vi "Window-Error message.vi"(8 "error in (no error)":errorcluster, 11 "Message":string) -> (0 "Error Out (no error)":errorcluster)   [LabVIEW 2020]
doc: "Use this template to create a dialog box with event handling."
uses:
  <vilib>/Utility/error.llb/DialogType.ctl
  miscelaneous/Error window positioning/Error window pos FGV states.ctl
  Global Variables/General Globals.vi
panel:
  out "Message":string
  in  "Close":bool
  in  "Vertical Stop Button":bool
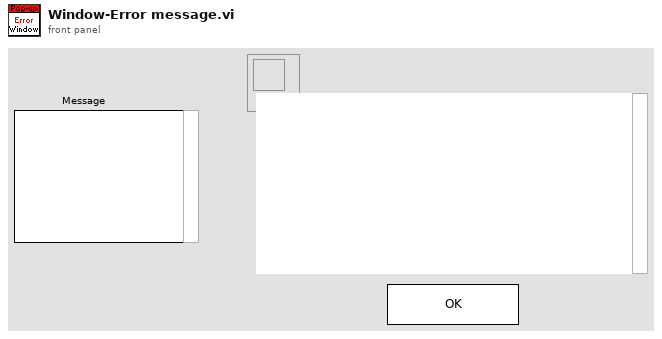
[diagram p1: front panel]
types:
  T1 = typedef "Error window pos FGV states.ctl" = enum16{"Read", "Window closed", "Window opened", "Reset"}
  T2 = typedef "DialogType.ctl" = u16
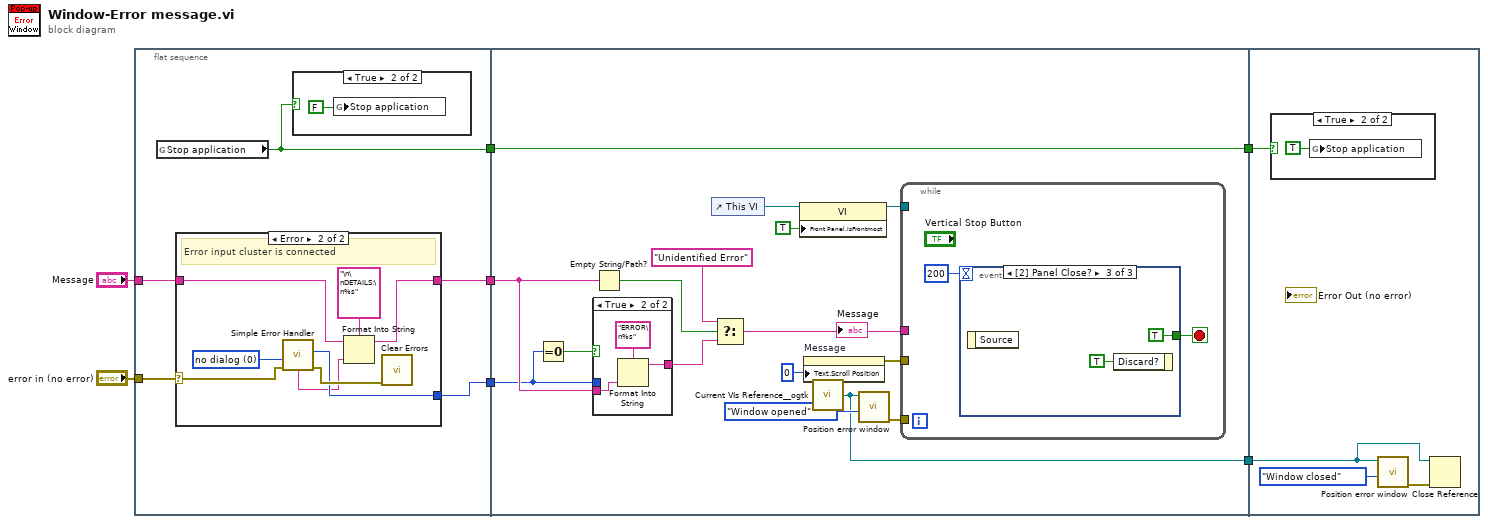
[diagram p0: block diagram]
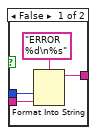
[diagram p4: hidden frame]
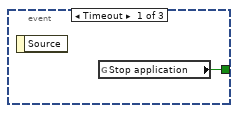
[diagram p5: hidden frame]
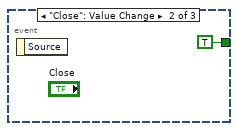
[diagram p6: hidden frame]
diagram:
  n1 = flat-sequence {
    tunnel: [w10] -> w7
    tunnel: [w9] -> w5
    tunnel: "Message" -> [w11]
    tunnel: "error in (no error)" -> [w12]
    tunnel: [w8] -> w2
    tunnel: w7 -> [w28]
    tunnel: [w32] -> w6
    tunnel: w5 -> [w32]
    tunnel: w2 -> [w26]
    tunnel: [w23] -> w1
    tunnel: w6 -> [w55]
    tunnel: w1 -> [w52]
    frame #0 {
      n2 = global read "General Globals.vi" "Stop application"() -> (w9:bool)
      n3 = case shown="Error" w12 {
        selector: w12 -> [_ w17]
        tunnel: w11 -> [w13 w15]
        tunnel: [w13 w18] -> w10
        tunnel: [_ w16] -> w8
        frame No Error {
          # "Error input cluster is not connected"
        }
        frame Error {
          w21 = T2 0 items=["no dialog", "OK message", "continue or stop message", "OK message + warnings", "continue/stop + warnings"] ("type of dialog (OK msg:1)")
          # "Error input cluster is connected"
          n4 = call <vilib>:"Simple Error Handler.vi"("type of dialog (OK msg:1)"=w21, "error in (no error)"=w17) -> ("code out"=w16:i32, "error out"=w19:errorcluster, "message"=w14:string)  [unwired: 3 in, 2 out]
          n5 = Format Into String(format string="\n\nDETAILS:\n%s", initial string=w15, w14) -> (resulting string=w18:string)  [unwired: 1 in, 1 out]
          n6 = call <vilib>:"Clear Errors.vi"("error in (no error)"=w19) -> ()  [unwired: 5 in, 2 out]
        }
      }
      n7 = case shown="True" w9 {
        frame False {
        }
        frame True {
          n8 = global write "General Globals.vi" "Stop application"(FALSE ("Quit?")) -> ()
        }
      }
    }
    frame #1 {
      n9 = Equal To 0?(x=w26) -> (x = 0?=w27:bool)
      n10 = case shown="True" w27 {
        tunnel: [w42 w45] -> w33
        tunnel: w28 -> [w41 w43]
        tunnel: w26 -> [w40 _]
        frame False {
          n11 = Format Into String(format string="ERROR %d\n%s", w40, w41) -> (resulting string=w42:string)  [unwired: 2 in, 1 out]
        }
        frame True {
          n12 = Format Into String(format string="ERROR\n%s", w43) -> (resulting string=w45:string)  [unwired: 2 in, 1 out]
        }
      }
      n13 = Empty String/Path?(string/path=w28) -> (empty?=w38:bool)
      n14 = control-ref of="This VI"() -> (w30:refnum<vi>)
      n15 = Select(t="Unidentified Error" ("String"), s=w38, f=w33) -> (s? t:f=w34:string)
      "Message" <- w34
      n16 = property on="Property Node" class="VI"(reference=w30, "Front Panel.IsFrontmost"=TRUE ("Front Panel Window:Is Frontmost")) -> (reference out=w29:refnum<vi>)  [unwired: 1 in, 1 out]
      n17 = property on="Message" class="Str"("Text.Scroll Position"=u32 0) -> (error out=w35:errorcluster)  [unwired: 2 in, 1 out]
      n18 = call <userlib>:"Current VIs Reference__ogtk.vi"() -> ("Current VI's reference"=w23:refnum<vi>)  [unwired: 5 in]
      n19 = call "Position error window.vi"("Function"=Error_window_pos_FGV_states."Window opened", "Error Window ref"=w23) -> ("error out"=w25:errorcluster)  [unwired: 9 in]
      n20 = while {
        tunnel: w34 -> [_]
        tunnel: w35 -> [_]
        tunnel: w29 -> [_]
        tunnel: w25 -> [_]
        stop <- w47 stop-if-true
        n21 = event shown="[2] Panel Close?" {
          selector: _ -> [_ _ _]
          dyn-events: _ -> [_ _ _]
          timeout: 200 -> [_ _ _]
          tunnel: [w48 TRUE ("Stop?") TRUE ("Stop?")] -> w47
          event Timeout {
            n22 = event-data() -> ()  [unwired: 1 in, 1 out]
            n23 = global read "General Globals.vi" "Stop application"() -> (w48:bool)
          }
          event "Close": Value Change {
            n24 = event-data() -> ()  [unwired: 1 in, 1 out]
          }
          event Panel Close? {
            n25 = event-data() -> ()  [unwired: 1 in, 1 out]
            n26 = event-data("Discard?"=TRUE) -> ()  [unwired: 1 in, 1 out]
          }
        }
      }
    }
    frame #2 {
      n27 = case shown="True" w55 {
        frame False {
        }
        frame True {
          n28 = global write "General Globals.vi" "Stop application"(TRUE ("Quit?")) -> ()
        }
      }
      n29 = call "Position error window.vi"("Function"=Error_window_pos_FGV_states."Window closed", "Error Window ref"=w52) -> ("error out"=w53:errorcluster)  [unwired: 9 in]
      n30 = Close Reference(reference=w52, error in (no error)=w53) -> ()  [unwired: 1 out]
    }
  }
